vi "InitDevices.vi"(8 "error in (no error)":errorcluster, 10 "Sensor Groups (false)":bool, 11 "config in":T3) -> (0 "error out":errorcluster, 2 "register trends":T1[](array[typedef]), 3 "config out":T3)   [LabVIEW 2017, in "ModbusMaster.lvlib"]
uses:
  <vilib>/addons/InsightCM/Devices/Shared/Common/ModbusMaster/ModbusMaster.lvlib
  <vilib>/addons/InsightCM/Devices/Shared/Common/ModbusMaster/controls/config.ctl
  <vilib>/addons/InsightCM/Devices/Shared/Common/ModbusMaster/controls/ModbusDevice.ctl
  <vilib>/Modbus/master/Modbus Master.lvclass
  <vilib>/addons/InsightCM/Devices/Shared/Common/ModbusMaster/controls/ModbusChannel.ctl
  <vilib>/addons/InsightCM/Devices/Shared/Common/ModbusMaster/controls/RegisterType.ctl
  <vilib>/addons/InsightCM/MessageBus/Base/controls/DataSource.ctl
  <vilib>/addons/InsightCM/MessageBus/Base/controls/KeyValuePair.ctl
  <vilib>/addons/InsightCM/Devices/Shared/Common/DataEventCreator/controls/RegisterTrendPoints.ctl
  <vilib>/addons/InsightCM/Devices/Shared/Common/DataEventCreator/controls/Registry_Trend.ctl
  <vilib>/addons/InsightCM/MessageBus/Base/controls/R2_Channel.ctl
  <vilib>/addons/InsightCM/MessageBus/Base/controls/Metric.ctl
  <vilib>/addons/InsightCM/Utilities/PropertyHelpers/PropertyHelpers.lvlib
  <vilib>/addons/InsightCM/Utilities/DeviceModelHelpers/DeviceModelHelpers.lvlib
  <vilib>/addons/InsightCM/Utilities/GlobalConfiguration/GlobalConfiguration.lvlib
  <vilib>/addons/InsightCM/Devices/Shared/Common/DataEventCreator/DataEventCreator.lvlib
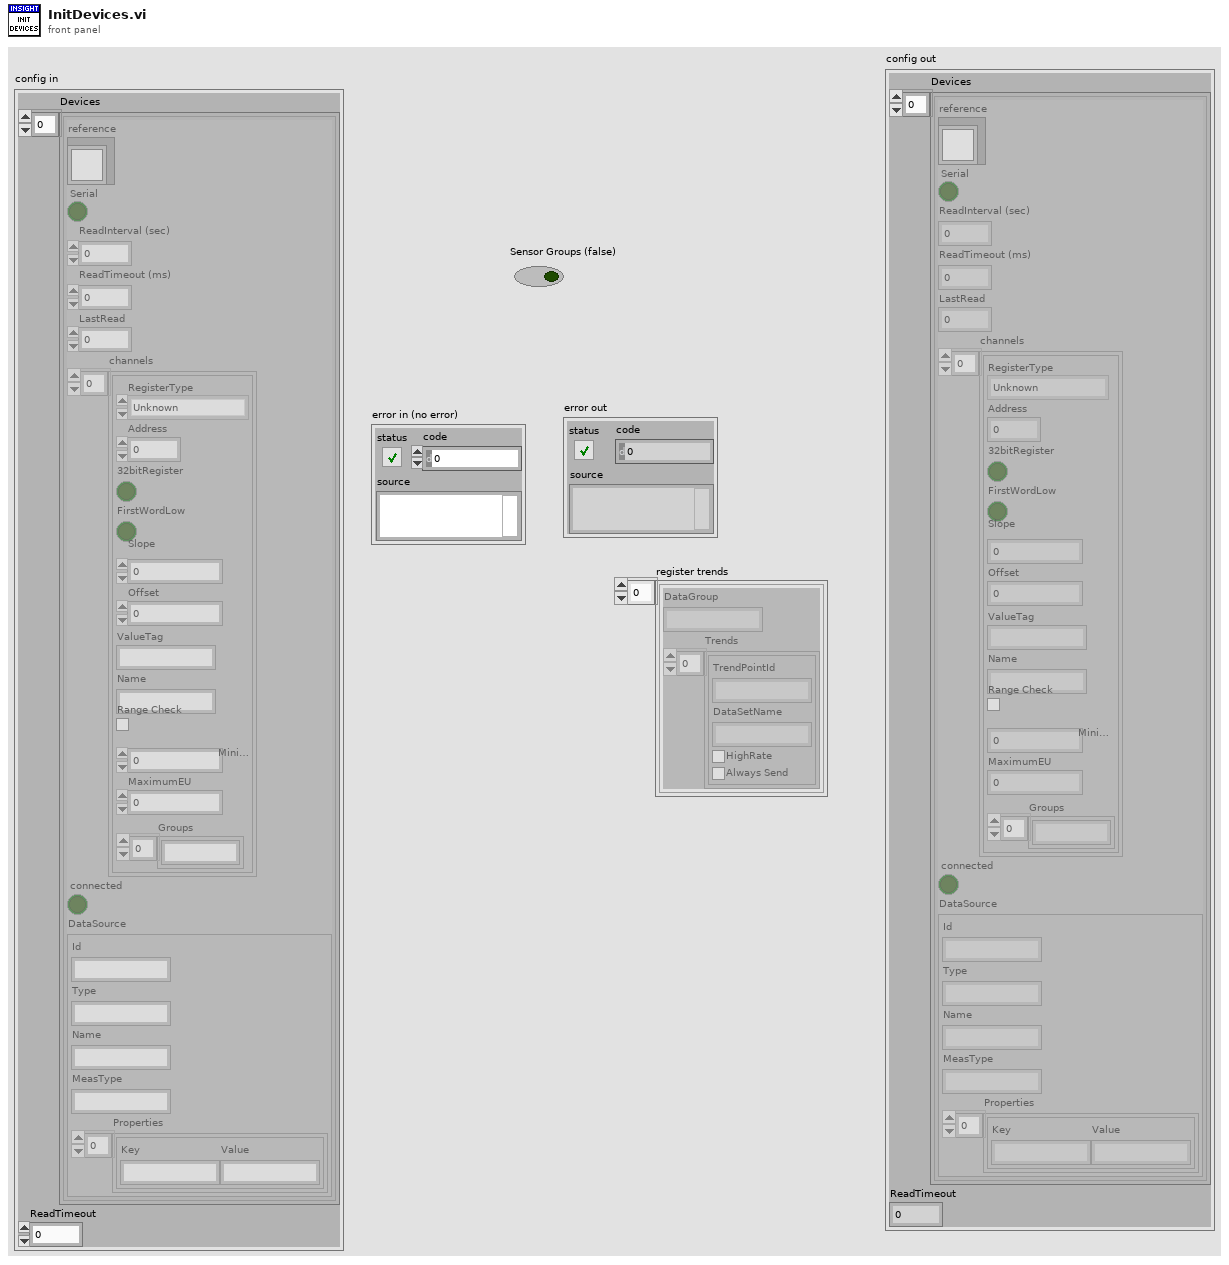
[diagram p1: front panel]
types:
  T1 = typedef "DataEventCreator.lvlib/RegisterTrendPoints.ctl" = cluster{"DataGroup":string, "Trends":T2[]}
  T2 = typedef "DataEventCreator.lvlib/Registry_Trend.ctl" = cluster{"TrendPointId":string, "DataSetName":string, "HighRate":bool, "Always Send":bool}
  T3 = typedef "ModbusMaster.lvlib/config.ctl" = cluster{"Devices":T4[], "ReadTimeout":i32}
  T4 = typedef "ModbusMaster.lvlib/ModbusDevice.ctl" = cluster{"reference":refnum<class "Modbus Master.lvclass">, "Serial":bool, "ReadInterval (sec)":dbl, "ReadTimeout (ms)":i32, "LastRead":dbl, "channels":T5[], "connected":bool, "DataSource":T7}
  T5 = typedef "ModbusMaster.lvlib/ModbusChannel.ctl" = cluster{"RegisterType":T6, "Address":i32, "32bitRegister":bool, "FirstWordLow":bool, "Slope":dbl, "Offset":dbl, "ValueTag":string, "Name":string, "Range Check":bool, "MinimumEU":dbl, "MaximumEU":dbl, "Groups":string[]}
  T6 = typedef "ModbusMaster.lvlib/RegisterType.ctl" = enum16{"Unknown", "Coil", "Discrete Input", "Holding Register", "Input Register"}
  T7 = typedef "DataSource.ctl" = cluster{"Id":string, "Type":string, "Name":string, "MeasType":string, "Properties":T8[]}
  T8 = typedef "KeyValuePair.ctl" = cluster{"Key":string, "Value":string}
  T9 = typedef "R2_DeviceModel.ctl" = cluster{"Device":T10, "Channels":T20[], "Tags":T22[]}
  T10 = typedef "R2_Device.ctl" = cluster{"Id":string, "Name":string, "DeviceType":string, "HardwareName":string, "IpAddress":string, "HardwareInfo":T8[], "ApplicationType":string, "ApplicationVersion":string, "EquipmentIds":string[], "ConfigurationVersion":string, "State":T11, "Properties":T8[], "DataGroups":T12[], "BurstModeTrigger":T16, "SensorGroups":T17[], "Endpoints":T18[]}
  T11 = typedef "DeviceState.ctl" = cluster{"Disabled":bool}
  T12 = typedef "R2_DataGroup.ctl" = cluster{"Name":string, "OperatingStates":T13[], "Properties":T8[], "EquipmentIds":string[], "AssetNodeId":string}
  T13 = typedef "OperatingState.ctl" = cluster{"Name":string, "Properties":T8[], "Triggers":T14[]}
  T14 = typedef "Trigger.ctl" = cluster{"Type":string, "Expression":string, "Conditions":T15[]}
  T15 = typedef "Condition.ctl" = cluster{"Source":string, "Type":string, "Operator":string, "CompareTo":string, "DwellSeconds":dbl}
  T16 = typedef "BurstModeTrigger.ctl" = cluster{"Trigger":T14, "SampleRate":string, "AcquisitionLength":string}
  T17 = typedef "DeviceSensorGroup.ctl" = cluster{"EquipId":string, "SensorGroupId":string}
  T18 = typedef "WirelessEndpoint.ctl" = cluster{"SerialNumber":string, "Properties":T8[], "Channels":T19[]}
  T19 = typedef "WirelessChannel.ctl" = cluster{"ChannelNumber":i32, "AssetId":string}
  T20 = typedef "R2_Channel.ctl" = cluster{"Id":string, "DeviceId":string, "Name":string, "ChannelType":string, "HardwareKey":string, "HardwareChannel":string, "DataGroup":string, "Keywords":string[], "EquipmentIds":string[], "Properties":T8[], "Metrics":T21[], "AssetNodeId":string, "MeasType":string, "AssetName":string}
  T21 = typedef "Metric.ctl" = cluster{"Id":string, "Name":string, "Unit":string, "Properties":T8[], "MetricDefinitionInstanceId":string}
  T22 = typedef "Tag.ctl" = cluster{"Id":string, "Path":string, "Name":string, "Datatype":string, "Props":T8[], "Keywords":string[]}
  T23 = typedef "AssetNode.ctl" = cluster{"Id":string, "Type":string, "Name":string, "ParentIds":string[], "State":T24, "MeasType":string, "Properties":T8[], "SensorGroups":T25[], "OperatingStates":T13[], "Metrics":T21[], "TrendAlarmRules":T27[], "References":T30[]}
  T24 = typedef "AssetState.ctl" = cluster{"Disabled":bool}
  T25 = typedef "AssetNodeSensorGroup.ctl" = cluster{"Id":string, "Type":string, "SensorIds":string[], "CollectionConfig":T26, "Properties":T8[]}
  T26 = typedef "WirelessCollectionConfig.ctl" = cluster{"GateCondition":T15, "CronString":string, "RetryIntervalMinutes":string, "MaxRetryAttempts":string}
  T27 = typedef "TrendAlarmRule.ctl" = cluster{"Id":string, "AssetNodeId":string, "TrendId":string, "Disabled":bool, "OperatingState":string, "Operator":string, "Hysteresis":dbl, "OnDelaySeconds":dbl, "OffDelaySeconds":dbl, "Levels":T28[], "Properties":T8[]}
  T28 = typedef "TrendAlarmLevel.ctl" = cluster{"Severity":i32, "CompareTo":dbl, "Actions":T29[]}
  T29 = typedef "AlarmAction.ctl" = cluster{"Type":string, "Props":T8[]}
  T30 = typedef "AssetNodeReference.ctl" = cluster{"NodeId":string, "Name":string}
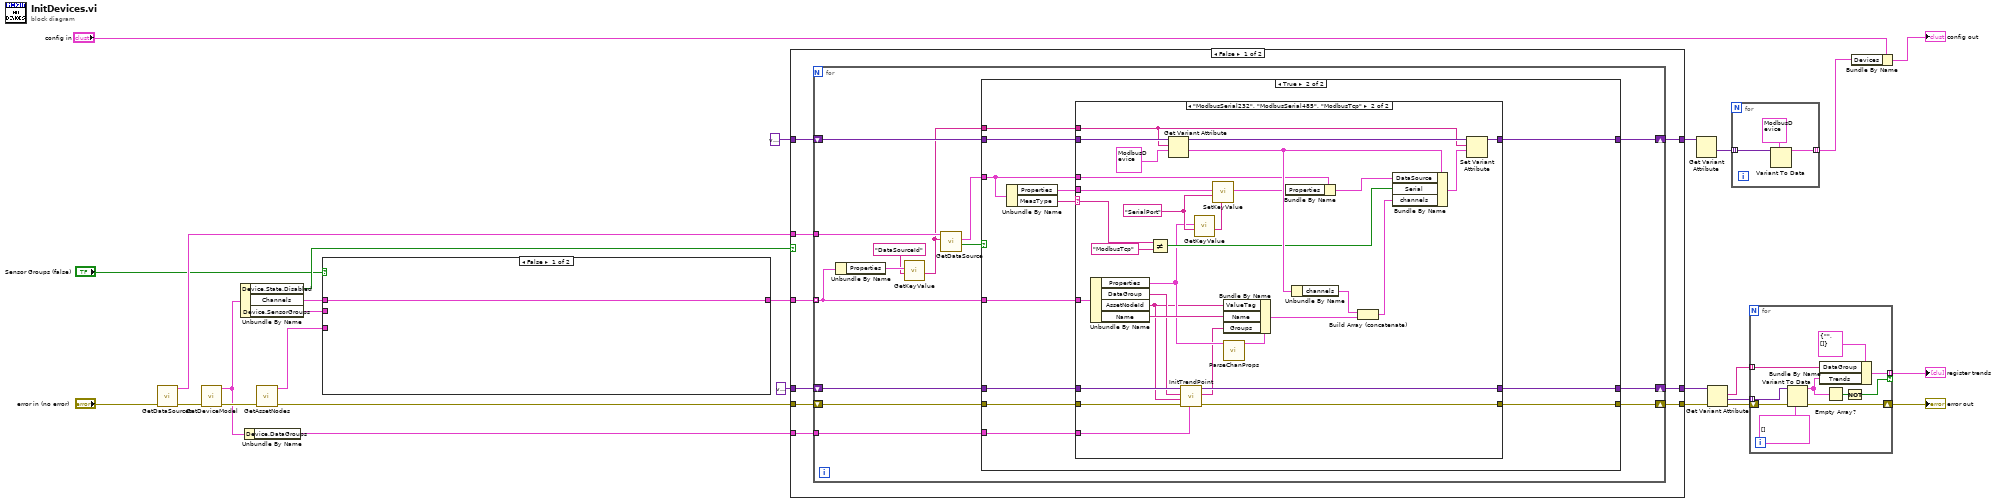
[diagram p0: block diagram]
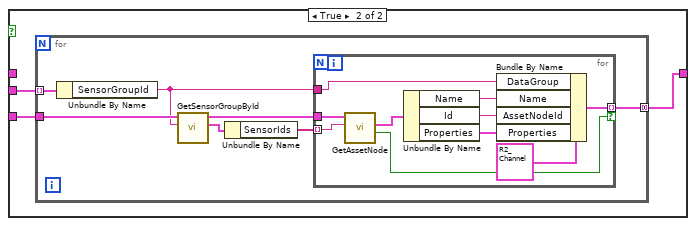
[diagram p2: hidden frame]
diagram:
  n1 = call <vilib>:"GetDataSources.vi"("error in (no error)"="error in (no error)") -> ("error out"=w18:errorcluster, "data sources"=w25:T7[])  [unwired: 8 in, 1 out]
  n2 = call <vilib>:"GetDeviceModel.vi"("error in (no error)"=w18) -> ("error out"=w9:errorcluster, "device model"=w7:T9)  [unwired: 8 in, 1 out]
  n3 = Unbundle By Name(w7) -> ("Device.State.Disabled"=w20:bool, "Channels"=w4:T20[], "Device.SensorGroups"=w1:T17[])
  n4 = Unbundle By Name(w7) -> ("Device.DataGroups"=w6:T12[])
  n5 = call <vilib>:"GetAssetNodes.vi"("error in (no error)"=w9) -> ("error out"=w8:errorcluster, "AssetNodes"=w2:T23[])  [unwired: 8 in, 1 out]
  n6 = case shown="False" "Sensor Groups (false)" {
    tunnel: [w28 w29] -> w5
    tunnel: w4 -> [w28 _]
    tunnel: w2 -> [_ w30]
    tunnel: w1 -> [_ w31]
    frame False {
    }
    frame True {
      n7 = for {
        tunnel: w31 -> [w38] mode=indexing
        tunnel: w30 -> [w37]
        tunnel: [w32] -> w29 mode=concatenating
        n8 = Unbundle By Name(w38) -> ("SensorGroupId"=w33:string)
        n9 = call <vilib>:"GetSensorGroupById.vi"("sensor group id"=w33, "asset nodes in"=w37) -> ("sensor group"=w36:T25, "asset nodes out"=w34:T23[])  [unwired: 7 in, 1 out]
        n10 = Unbundle By Name(w36) -> ("SensorIds"=w35:string[])
        n11 = for {
          tunnel: w35 -> [w47] mode=indexing
          tunnel: w34 -> [w48]
          tunnel: w33 -> [w40]
          tunnel: [w42] -> w32 mode=indexing if=w41
          n12 = call <vilib>:"GetAssetNode.vi"("node id"=w47, "nodes in"=w48) -> ("found"=w41:bool, "AssetNode"=w44:T23)  [unwired: 7 in, 1 out]
          n13 = Unbundle By Name(w44) -> ("Name"=w39:string, "Id"=w46:string, "Properties"=w45:T8[])
          n14 = Bundle By Name(cluster=T20 {"Id"="", "DeviceId"="", "Name"="", "ChannelType"="", "HardwareKey"="", "HardwareChannel"="", "DataGroup"="", "Keywords"=[], "EquipmentIds"=[], "Properties"=[], "Metrics"=[], "AssetNodeId"="", "MeasType"="", "AssetName"=""} ("ChannelModel"), "DataGroup"=w40, "Name"=w39, "AssetNodeId"=w46, "Properties"=w45) -> (w42:T20)
        }
      }
    }
  }
  n15 = case shown="False" w20 {
    tunnel: w25 -> [w57 _]
    tunnel: w5 -> [w54 _]
    tunnel: variant -> [w56 w122]
    tunnel: [w55 w122] -> w22
    tunnel: [w53 w120] -> w13
    tunnel: [w52 w121] -> w12
    tunnel: w8 -> [w51 w120]
    tunnel: variant ("data group map") -> [w50 w121]
    tunnel: w6 -> [w49 _]
    frame False {
      n16 = for {
        tunnel: w54 -> [w68] mode=indexing
        shift-right: [w71] -> w55
        shift-left: w56 -> [w70]
        tunnel: w57 -> [w69]
        shift-right: [w62] -> w53
        shift-left: w51 -> [w59]
        shift-right: [w61] -> w52
        shift-left: w50 -> [w60]
        tunnel: w49 -> [w58]
        n17 = Unbundle By Name(w68) -> ("Properties"=w67:T8[])
        n18 = call <vilib>:"GetKeyValue.vi"("key"="DataSourceId", "key value pairs"=w67) -> ("value"=w63:string)  [unwired: 7 in, 2 out]
        n19 = call <vilib>:"GetDataSource.vi"("data source id"=w63, "data sources in"=w69) -> ("found"=w65:bool, "DataSource"=w64:T7)  [unwired: 7 in, 1 out]
        n20 = case shown="True" w65 {
          tunnel: [w74 w85] -> w71
          tunnel: w70 -> [w74 w86]
          tunnel: w64 -> [_ w82]
          tunnel: w63 -> [_ w84]
          tunnel: w68 -> [_ w83]
          tunnel: [w72 w79] -> w62
          tunnel: [w73 w78] -> w61
          tunnel: w60 -> [w73 w77]
          tunnel: w59 -> [w72 w76]
          tunnel: w58 -> [_ w75]
          frame False {
          }
          frame True {
            n21 = Unbundle By Name(w82) -> ("Properties"=w80:T8[], "MeasType"=w81:string)
            n22 = case shown="\"ModbusSerial232\", \"ModbusSerial485\", \"ModbusTcp\"" w81 {
              selector: w81 -> [_ w100]
              tunnel: w86 -> [w89 w118]
              tunnel: [w89 w117] -> w85
              tunnel: w84 -> [_ w115]
              tunnel: w83 -> [_ w112]
              tunnel: w82 -> [_ w107]
              tunnel: w80 -> [_ w101]
              tunnel: [w87 w95] -> w79
              tunnel: [w88 w97] -> w78
              tunnel: w77 -> [w88 w94]
              tunnel: w76 -> [w87 w96]
              tunnel: w75 -> [_ w90]
              frame Default {
              }
              frame "ModbusSerial232", "ModbusSerial485", "ModbusTcp" {
                w109 = "SerialPort" ("key")
                n23 = Unbundle By Name(w112) -> ("Properties"=w99:T8[], "DataGroup"=w93:string, "AssetNodeId"=w92:string, "Name"=w111:string)
                n24 = Not Equal?(x=w100, y="ModbusTcp" ("x")) -> (x != y?=w102:bool)
                n25 = Get Variant Attribute(Variant=w118, name=w115, default value (empty Variant)=T4 {"reference"=refnum, "Serial"=FALSE, "ReadInterval (sec)"=0.0, "ReadTimeout (ms)"=0, "LastRead"=0.0, "channels"=[], "connected"=FALSE, "DataSource"={"Id"="", "Type"="", "Name"="", "MeasType"="", "Properties"=[]}} ("device")) -> (value=w116:T4)  [unwired: 1 in, 3 out]
                n26 = call <vilib>:"InitTrendPoint.vi"("DataGroups"=w90, "error in (no error)"=w96, "AssetNodeId"=w92, "DataGroup"=w93, "trend registrations in"=w94) -> ("error out"=w95:errorcluster, "groups"=w91:string[], "trend registrations out"=w97:variant)  [unwired: 4 in]
                n27 = call <vilib>:"GetKeyValue.vi"("key"=w109, "key value pairs"=w99) -> ("value"=w108:string)  [unwired: 7 in, 2 out]
                n28 = call <vilib>:"SetKeyValue.vi"("value"=w108, "key"=w109, "key value pairs"=w101) -> ("key value pairs out"=w106:T8[])  [unwired: 8 in]
                n29 = call <vilib>:"ParseChanProps.vi"("properties"=w99) -> ("channel"=w98:T5)  [unwired: 9 in, 1 out]
                n30 = Bundle By Name(cluster=w98, "ValueTag"=w92, "Name"=w111, "Groups"=w91) -> (w113:T5)
                n31 = Bundle By Name(cluster=w107, "Properties"=w106) -> (w105:T7)
                n32 = Unbundle By Name(w116) -> ("channels"=w114:T5[])
                n33 = Build Array (concatenate)(w114, w113) -> (w110:T5[])
                n34 = Bundle By Name(cluster=w116, "DataSource"=w105, "Serial"=w102, "channels"=w110) -> (w104:T4)
                n35 = Set Variant Attribute(Variant=w118, name=w115, value=w104) -> (Variant out=w117:variant)  [unwired: 1 in, 2 out]
              }
            }
          }
        }
      }
    }
    frame True {
    }
  }
  n36 = Get Variant Attribute(Variant=w22) -> (values=w21:variant[])  [unwired: 3 in, 3 out]
  n37 = Get Variant Attribute(Variant=w12, error in=w13) -> (names=w14:string[], values=w16:variant[], error out=w15:errorcluster)  [unwired: 2 in, 1 out]
  n38 = for {
    tunnel: w21 -> [w125] mode=indexing
    tunnel: [w123] -> w19 mode=indexing
    n39 = Variant To Data(type=T4 {"reference"=refnum, "Serial"=FALSE, "ReadInterval (sec)"=0.0, "ReadTimeout (ms)"=0, "LastRead"=0.0, "channels"=[], "connected"=FALSE, "DataSource"={"Id"="", "Type"="", "Name"="", "MeasType"="", "Properties"=[]}} ("device"), Variant=w125) -> (data=w123:T4)  [unwired: 1 in, 1 out]
  }
  n40 = for {
    tunnel: w16 -> [w130] mode=indexing
    tunnel: [w133] -> w17 mode=indexing if=w132
    tunnel: w14 -> [w128] mode=indexing
    shift-right: [w126] -> w10
    shift-left: w15 -> [w127]
    n41 = Variant To Data(error in=w127, type=T2[] [], Variant=w130) -> (data=w129:T2[], error out=w126:errorcluster)
    n42 = Bundle By Name(cluster=T1 {"DataGroup"="", "Trends"=[]} ("register trend"), "DataGroup"=w128, "Trends"=w129) -> (w133:T1)
    n43 = Empty Array?(array=w129) -> (empty?=w134:bool)
    n44 = Not(x=w134) -> (.not. x?=w132:bool)
  }
  "error out" <- w10
  "register trends" <- w17
  n45 = Bundle By Name(cluster="config in", "Devices"=w19) -> (→"config out":T3)
